vi "NewTCPServerDialog.vi"() -> (16 "执行完成":bool)   [LabVIEW 2019]
uses:
  02 Mode/TCPServerMode/TCPServerClass.lvclass
panel:
  in  "取消":bool
  in  "确认":bool
  in  "服务端识别":cluster{"本机IP":string, "本机端口":u16}={"本机IP"="127.0.0.1", "本机端口"=4001}
  in  "停止":bool
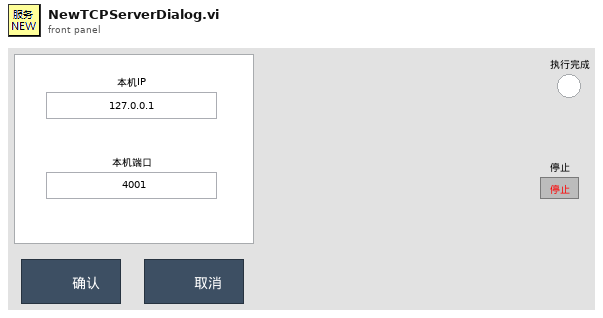
[diagram p1: front panel]
types:
  T1 = map{string, refnum<class "TCPServerClass.lvclass">}
  T2 = cluster{"IP:Port":string, "TCPServerClass 输出":refnum<class "TCPServerClass.lvclass">}
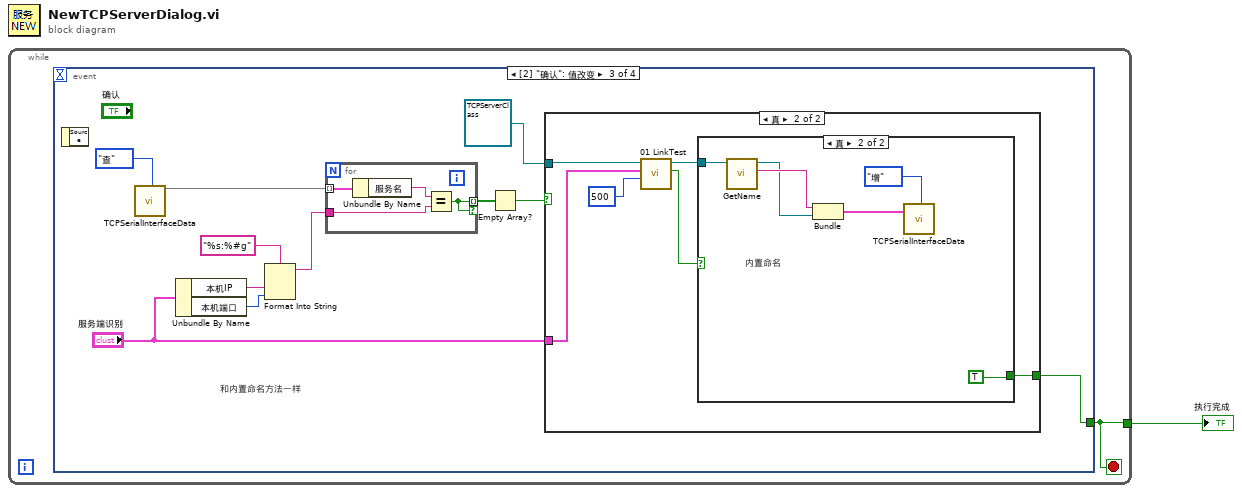
[diagram p0: block diagram]
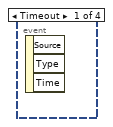
[diagram p2: hidden frame]
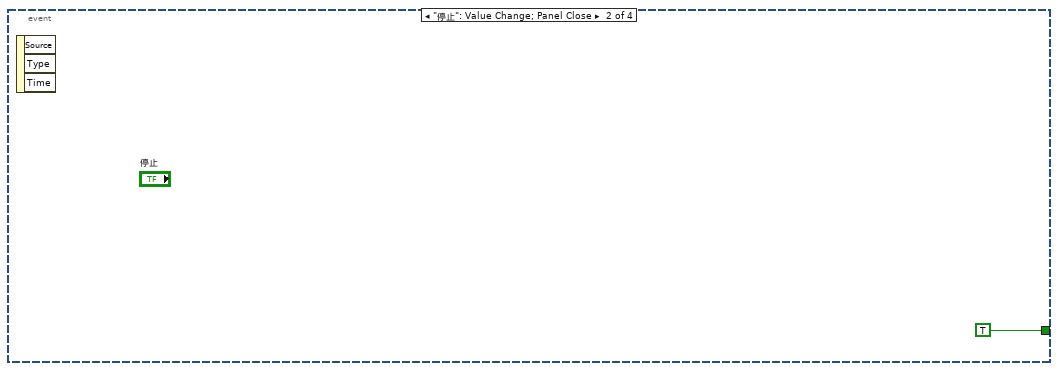
[diagram p3: hidden frame]
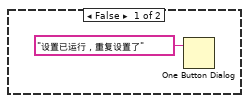
[diagram p4: hidden frame]
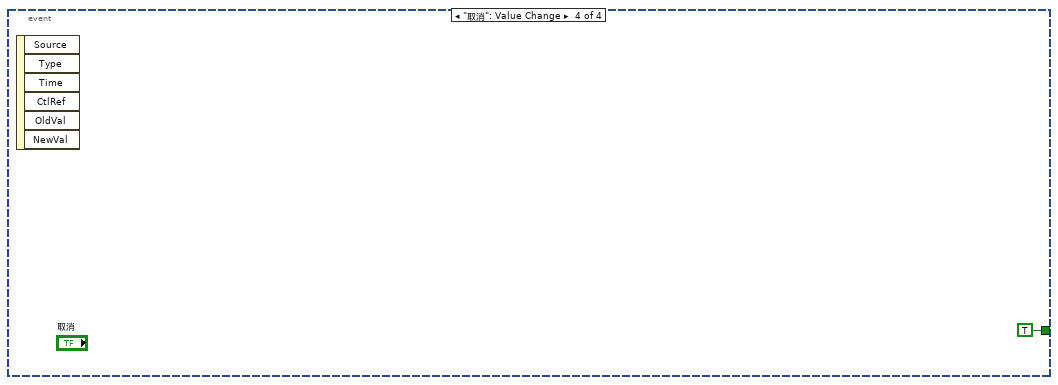
[diagram p6: hidden frame]
diagram:
  n1 = while {
    tunnel: [w2] -> w1
    stop <- w2 stop-if-true
    n2 = event shown="[2] \"确认\": 值改变" {
      selector: _ -> [_ _ _ _]
      dyn-events: _ -> [_ _ _ _]
      timeout: _ -> [_ _ _ _]
      tunnel: [_ TRUE ("停止") w5 TRUE ("停止")] -> w2
      event Timeout {
        n3 = event-data() -> ()  [unwired: 1 in, 3 out]
      }
      event "停止": Value Change; Panel Close {
        n4 = event-data() -> ()  [unwired: 1 in, 3 out]
      }
      event "确认": Value Change {
        # "和内置命名方法一样"
        n5 = event-data() -> ()  [unwired: 1 in, 1 out]
        n6 = call "TCPSerialInterfaceData.vi"("客服接口枚举"=enum16{"ini", "增", "删", "查", "改", "腾笼换鸟"}."查") -> ("服务表"=w11:T1)  [unwired: 17 in, 1 out]
        n7 = Unbundle By Name("服务端识别") -> ("本机IP"=w13:string, "本机端口"=w12:u16)
        n8 = Format Into String(format string="%s:%#g" ("格式字符串"), w13, w12) -> (resulting string=w10:string)  [unwired: 2 in, 1 out]
        n9 = for {
          tunnel: w11 -> [w31] mode=indexing
          tunnel: w10 -> [w30]
          tunnel: [w29] -> w9 mode=indexing if=w29
          n10 = Unbundle By Name(w31) -> ("服务名"=w28:string)
          n11 = Equal?(x=w28, y=w30) -> (x = y?=w29:bool)
        }
        n12 = Empty Array?(array=w9) -> (empty?=w8:bool)
        n13 = case shown="真" w8 {
          tunnel: refnum<class "TCPServerClass.lvclass"> refnum ("服务类") -> [_ w21]
          tunnel: "服务端识别" -> [_ w20]
          tunnel: [_ w16] -> w5
          frame False {
            n14 = One Button Dialog(message="设置已运行，重复设置了" ("消息")) -> ()  [unwired: 1 in, 1 out]
          }
          frame True {
            n15 = call-dynamic "01 LinkTest.vi"("超时毫秒"=500, "服务端识别"=w20, "TCPServerClass 输入"=w21) -> ("成功？"=w18:bool, "TCPServerClass 输出"=w17:refnum<class "TCPServerClass.lvclass">)  [unwired: 6 in, 1 out]
            n16 = case shown="真" w18 {
              tunnel: w17 -> [_ w27]
              tunnel: [_ TRUE] -> w16
              frame False {
                # "提示在侦听创建里\n失败警告弹窗"
              }
              frame True {
                # "内置命名"
                n17 = call-dynamic "GetName.vi"("TCPServerClass 输入"=w27) -> ("IP:Port"=w26:string, "TCPServerClass 输出"=w25:refnum<class "TCPServerClass.lvclass">)  [unwired: 8 in, 1 out]
                n18 = Bundle("IP:Port"=w26, "TCPServerClass 输出"=w25) -> (w24:T2)  [unwired: 1 in]
                n19 = call "TCPSerialInterfaceData.vi"("信息"=w24, "客服接口枚举"=enum16{"ini", "增", "删", "查", "改", "腾笼换鸟"}."增") -> ()  [unwired: 16 in, 2 out]
              }
            }
          }
        }
      }
      event "取消": Value Change {
        n20 = event-data() -> ()  [unwired: 1 in, 6 out]
      }
    }
  }
  "执行完成" <- w1
